vi "myRIO_BRig_Host_endExp_storeFiles.vi"(0 "input_filePath":path) -> (4 "output_IdataBlock":bool, 6 "output_IdataCurrent":bool, 8 "output_IdataExp":bool, 10 "output_IdataLC":bool, 13 "output_IdataTrial":bool, 14 "output_IdataMTrig":bool, 15 "output_IdataLick":bool)   [LabVIEW 2014]
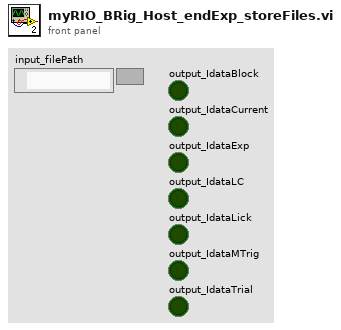
[diagram p1: front panel]
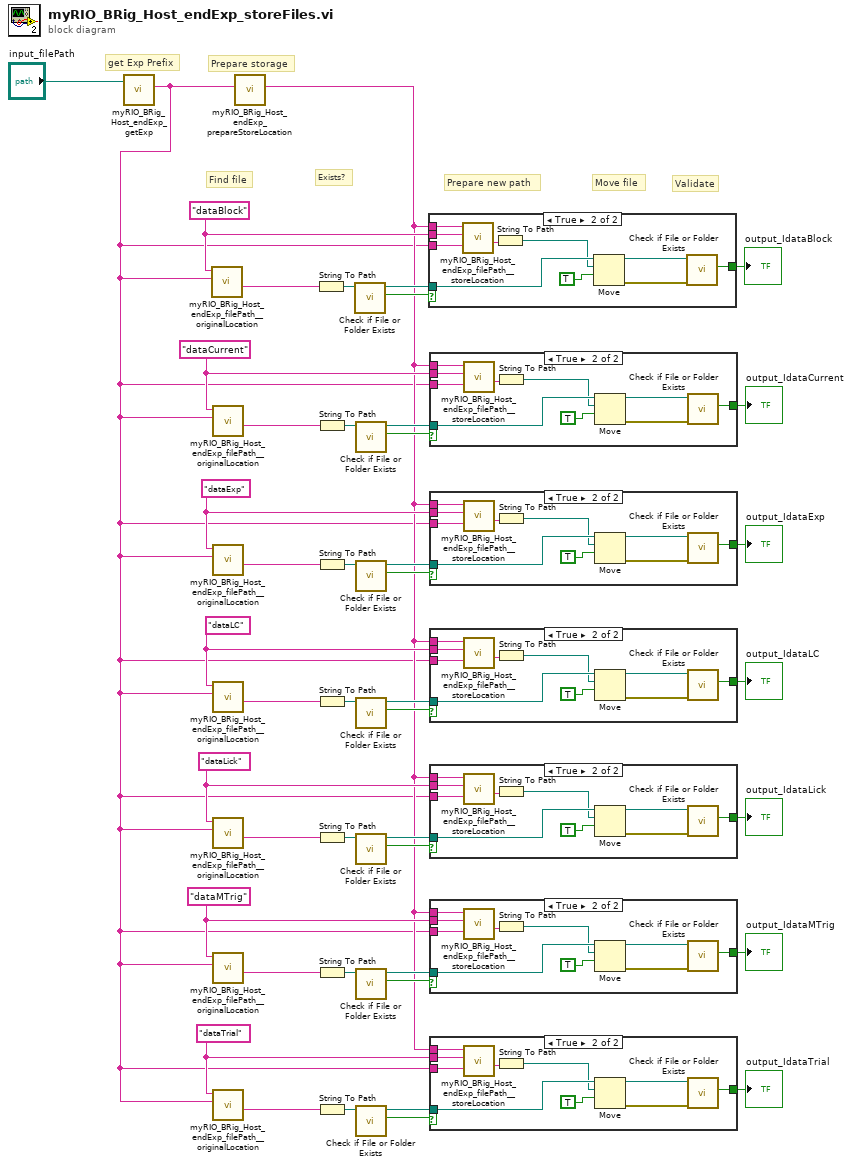
[diagram p0: block diagram]
diagram:
  w5 = "dataTrial" ("input_fileName")
  w11 = "dataMTrig" ("input_fileName")
  w17 = "dataLick" ("input_fileName")
  w23 = "dataLC" ("input_fileName")
  w29 = "dataExp" ("input_fileName")
  w35 = "dataCurrent" ("input_fileName")
  w41 = "dataBlock" ("input_fileName")
  # "Validate"
  # "Move file"
  # "Prepare new path"
  # "Exists?"
  # "Find file"
  # "Prepare storage"
  # "get Exp Prefix"
  n1 = call "myRIO_BRig_Host_endExp_getExp.vi"("input_filePath"="input_filePath") -> ("output_expPrefix"=w1:string)  [unwired: 10 in]
  n2 = call "myRIO_BRig_Host_endExp_filePath__originalLocation.vi"("input_expPrefix"=w1, "input_fileName"=w41) -> ("output_filePath"=w43:string)  [unwired: 9 in]
  n3 = call "myRIO_BRig_Host_endExp_filePath__originalLocation.vi"("input_expPrefix"=w1, "input_fileName"=w35) -> ("output_filePath"=w37:string)  [unwired: 9 in]
  n4 = call "myRIO_BRig_Host_endExp_filePath__originalLocation.vi"("input_expPrefix"=w1, "input_fileName"=w29) -> ("output_filePath"=w31:string)  [unwired: 9 in]
  n5 = call "myRIO_BRig_Host_endExp_filePath__originalLocation.vi"("input_expPrefix"=w1, "input_fileName"=w23) -> ("output_filePath"=w25:string)  [unwired: 9 in]
  n6 = call "myRIO_BRig_Host_endExp_filePath__originalLocation.vi"("input_expPrefix"=w1, "input_fileName"=w17) -> ("output_filePath"=w19:string)  [unwired: 9 in]
  n7 = call "myRIO_BRig_Host_endExp_filePath__originalLocation.vi"("input_expPrefix"=w1, "input_fileName"=w11) -> ("output_filePath"=w13:string)  [unwired: 9 in]
  n8 = call "myRIO_BRig_Host_endExp_filePath__originalLocation.vi"("input_expPrefix"=w1, "input_fileName"=w5) -> ("output_filePath"=w7:string)  [unwired: 9 in]
  n9 = call "myRIO_BRig_Host_endExp_prepareStoreLocation.vi"("input_expPrefix"=w1) -> ("output_folderPath"=w2:string)  [unwired: 10 in]
  n10 = String To Path(string=w43) -> (path=w44:path)
  n11 = String To Path(string=w37) -> (path=w38:path)
  n12 = String To Path(string=w31) -> (path=w32:path)
  n13 = String To Path(string=w25) -> (path=w26:path)
  n14 = String To Path(string=w19) -> (path=w20:path)
  n15 = String To Path(string=w13) -> (path=w14:path)
  n16 = String To Path(string=w7) -> (path=w8:path)
  n17 = call <vilib>:"Check if File or Folder Exists.vi"("path"=w44) -> ("file or folder exists?"=w42:bool, "dup path"=w40:path)  [unwired: 8 in, 1 out]
  n18 = call <vilib>:"Check if File or Folder Exists.vi"("path"=w38) -> ("file or folder exists?"=w36:bool, "dup path"=w34:path)  [unwired: 8 in, 1 out]
  n19 = call <vilib>:"Check if File or Folder Exists.vi"("path"=w32) -> ("file or folder exists?"=w30:bool, "dup path"=w28:path)  [unwired: 8 in, 1 out]
  n20 = call <vilib>:"Check if File or Folder Exists.vi"("path"=w26) -> ("file or folder exists?"=w24:bool, "dup path"=w22:path)  [unwired: 8 in, 1 out]
  n21 = call <vilib>:"Check if File or Folder Exists.vi"("path"=w20) -> ("file or folder exists?"=w18:bool, "dup path"=w16:path)  [unwired: 8 in, 1 out]
  n22 = call <vilib>:"Check if File or Folder Exists.vi"("path"=w14) -> ("file or folder exists?"=w12:bool, "dup path"=w10:path)  [unwired: 8 in, 1 out]
  n23 = call <vilib>:"Check if File or Folder Exists.vi"("path"=w8) -> ("file or folder exists?"=w6:bool, "dup path"=w4:path)  [unwired: 8 in, 1 out]
  n24 = case shown="True" w42 {
    tunnel: w41 -> [_ w54]
    tunnel: w1 -> [_ w55]
    tunnel: w40 -> [_ w47]
    tunnel: w2 -> [_ w53]
    tunnel: [_ w48] -> w39
    frame False {
    }
    frame True {
      n25 = call "myRIO_BRig_Host_endExp_filePath__storeLocation.vi"("input_expPrefix"=w55, "input_fileName"=w54, "input_filePath_storage"=w53) -> ("output_filePath"=w52:string)  [unwired: 8 in]
      n26 = String To Path(string=w52) -> (path=w46:path)
      n27 = Move(source path=w47, 9:TRUE ("overwrite (F)"), 10:w46) -> (error out=w49:errorcluster, 3:w50:path)  [unwired: 2 in, 1 out]
      n28 = call <vilib>:"Check if File or Folder Exists.vi"("error in (no error)"=w49, "path"=w50) -> ("file or folder exists?"=w48:bool)  [unwired: 7 in, 2 out]
    }
  }
  "output_IdataBlock" <- w39
  n29 = case shown="True" w36 {
    tunnel: w35 -> [_ w64]
    tunnel: w1 -> [_ w65]
    tunnel: w34 -> [_ w57]
    tunnel: w2 -> [_ w63]
    tunnel: [_ w58] -> w33
    frame False {
    }
    frame True {
      n30 = call "myRIO_BRig_Host_endExp_filePath__storeLocation.vi"("input_expPrefix"=w65, "input_fileName"=w64, "input_filePath_storage"=w63) -> ("output_filePath"=w62:string)  [unwired: 8 in]
      n31 = String To Path(string=w62) -> (path=w56:path)
      n32 = Move(source path=w57, 9:TRUE ("overwrite (F)"), 10:w56) -> (error out=w59:errorcluster, 3:w60:path)  [unwired: 2 in, 1 out]
      n33 = call <vilib>:"Check if File or Folder Exists.vi"("error in (no error)"=w59, "path"=w60) -> ("file or folder exists?"=w58:bool)  [unwired: 7 in, 2 out]
    }
  }
  "output_IdataCurrent" <- w33
  n34 = case shown="True" w30 {
    tunnel: w29 -> [_ w74]
    tunnel: w1 -> [_ w75]
    tunnel: w28 -> [_ w67]
    tunnel: w2 -> [_ w73]
    tunnel: [_ w68] -> w27
    frame False {
    }
    frame True {
      n35 = call "myRIO_BRig_Host_endExp_filePath__storeLocation.vi"("input_expPrefix"=w75, "input_fileName"=w74, "input_filePath_storage"=w73) -> ("output_filePath"=w72:string)  [unwired: 8 in]
      n36 = String To Path(string=w72) -> (path=w66:path)
      n37 = Move(source path=w67, 9:TRUE ("overwrite (F)"), 10:w66) -> (error out=w69:errorcluster, 3:w70:path)  [unwired: 2 in, 1 out]
      n38 = call <vilib>:"Check if File or Folder Exists.vi"("error in (no error)"=w69, "path"=w70) -> ("file or folder exists?"=w68:bool)  [unwired: 7 in, 2 out]
    }
  }
  "output_IdataExp" <- w27
  n39 = case shown="True" w24 {
    tunnel: w23 -> [_ w84]
    tunnel: w1 -> [_ w85]
    tunnel: w22 -> [_ w77]
    tunnel: w2 -> [_ w83]
    tunnel: [_ w78] -> w21
    frame False {
    }
    frame True {
      n40 = call "myRIO_BRig_Host_endExp_filePath__storeLocation.vi"("input_expPrefix"=w85, "input_fileName"=w84, "input_filePath_storage"=w83) -> ("output_filePath"=w82:string)  [unwired: 8 in]
      n41 = String To Path(string=w82) -> (path=w76:path)
      n42 = Move(source path=w77, 9:TRUE ("overwrite (F)"), 10:w76) -> (error out=w79:errorcluster, 3:w80:path)  [unwired: 2 in, 1 out]
      n43 = call <vilib>:"Check if File or Folder Exists.vi"("error in (no error)"=w79, "path"=w80) -> ("file or folder exists?"=w78:bool)  [unwired: 7 in, 2 out]
    }
  }
  "output_IdataLC" <- w21
  n44 = case shown="True" w18 {
    tunnel: w17 -> [_ w94]
    tunnel: w1 -> [_ w95]
    tunnel: w16 -> [_ w87]
    tunnel: w2 -> [_ w93]
    tunnel: [_ w88] -> w15
    frame False {
    }
    frame True {
      n45 = call "myRIO_BRig_Host_endExp_filePath__storeLocation.vi"("input_expPrefix"=w95, "input_fileName"=w94, "input_filePath_storage"=w93) -> ("output_filePath"=w92:string)  [unwired: 8 in]
      n46 = String To Path(string=w92) -> (path=w86:path)
      n47 = Move(source path=w87, 9:TRUE ("overwrite (F)"), 10:w86) -> (error out=w89:errorcluster, 3:w90:path)  [unwired: 2 in, 1 out]
      n48 = call <vilib>:"Check if File or Folder Exists.vi"("error in (no error)"=w89, "path"=w90) -> ("file or folder exists?"=w88:bool)  [unwired: 7 in, 2 out]
    }
  }
  "output_IdataLick" <- w15
  n49 = case shown="True" w12 {
    tunnel: w11 -> [_ w104]
    tunnel: w1 -> [_ w105]
    tunnel: w10 -> [_ w97]
    tunnel: w2 -> [_ w103]
    tunnel: [_ w98] -> w9
    frame False {
    }
    frame True {
      n50 = call "myRIO_BRig_Host_endExp_filePath__storeLocation.vi"("input_expPrefix"=w105, "input_fileName"=w104, "input_filePath_storage"=w103) -> ("output_filePath"=w102:string)  [unwired: 8 in]
      n51 = String To Path(string=w102) -> (path=w96:path)
      n52 = Move(source path=w97, 9:TRUE ("overwrite (F)"), 10:w96) -> (error out=w99:errorcluster, 3:w100:path)  [unwired: 2 in, 1 out]
      n53 = call <vilib>:"Check if File or Folder Exists.vi"("error in (no error)"=w99, "path"=w100) -> ("file or folder exists?"=w98:bool)  [unwired: 7 in, 2 out]
    }
  }
  "output_IdataMTrig" <- w9
  n54 = case shown="True" w6 {
    tunnel: w5 -> [_ w114]
    tunnel: w1 -> [_ w115]
    tunnel: w4 -> [_ w107]
    tunnel: w2 -> [_ w113]
    tunnel: [_ w108] -> w3
    frame False {
    }
    frame True {
      n55 = call "myRIO_BRig_Host_endExp_filePath__storeLocation.vi"("input_expPrefix"=w115, "input_fileName"=w114, "input_filePath_storage"=w113) -> ("output_filePath"=w112:string)  [unwired: 8 in]
      n56 = String To Path(string=w112) -> (path=w106:path)
      n57 = Move(source path=w107, 9:TRUE ("overwrite (F)"), 10:w106) -> (error out=w109:errorcluster, 3:w110:path)  [unwired: 2 in, 1 out]
      n58 = call <vilib>:"Check if File or Folder Exists.vi"("error in (no error)"=w109, "path"=w110) -> ("file or folder exists?"=w108:bool)  [unwired: 7 in, 2 out]
    }
  }
  "output_IdataTrial" <- w3
